vi "ROS_ParseMsg_r2.vi"(8 "Msg Package Path (blank)":path, 9 "Message Type":string, 11 "msg in":string) -> (1 "data":variant[](array[variant]), 3 "msg out":string)   [LabVIEW 2016]
doc: "Parses a ROS message based on the Message Type. Message Type must be a valid .txt file in the RosMessages directory."
uses:
  std_msgs/subs/parse_bool_scalar.vi
  std_msgs/subs/parse_i8_scalar.vi
  std_msgs/subs/parse_u8_scalar.vi
  std_msgs/subs/parse_i16_scalar.vi
  std_msgs/subs/parse_u16_scalar.vi
  std_msgs/subs/parse_i32_scalar.vi
  std_msgs/subs/parse_u32_scalar.vi
  std_msgs/subs/parse_i64_scalar.vi
  std_msgs/subs/parse_u64_scalar.vi
  std_msgs/subs/parse_float32_scalar.vi
  std_msgs/subs/parse_float64_scalar.vi
  std_msgs/subs/parse_string_scalar.vi
  std_msgs/subs/parse_time_scalar.vi
  std_msgs/subs/parse_duration_scalar.vi
panel:
  out "Data Types":string[](array[string])
  out "Data Names":string[](array[string])
  out "msg def":string
  out "Comments":string[](array[string])
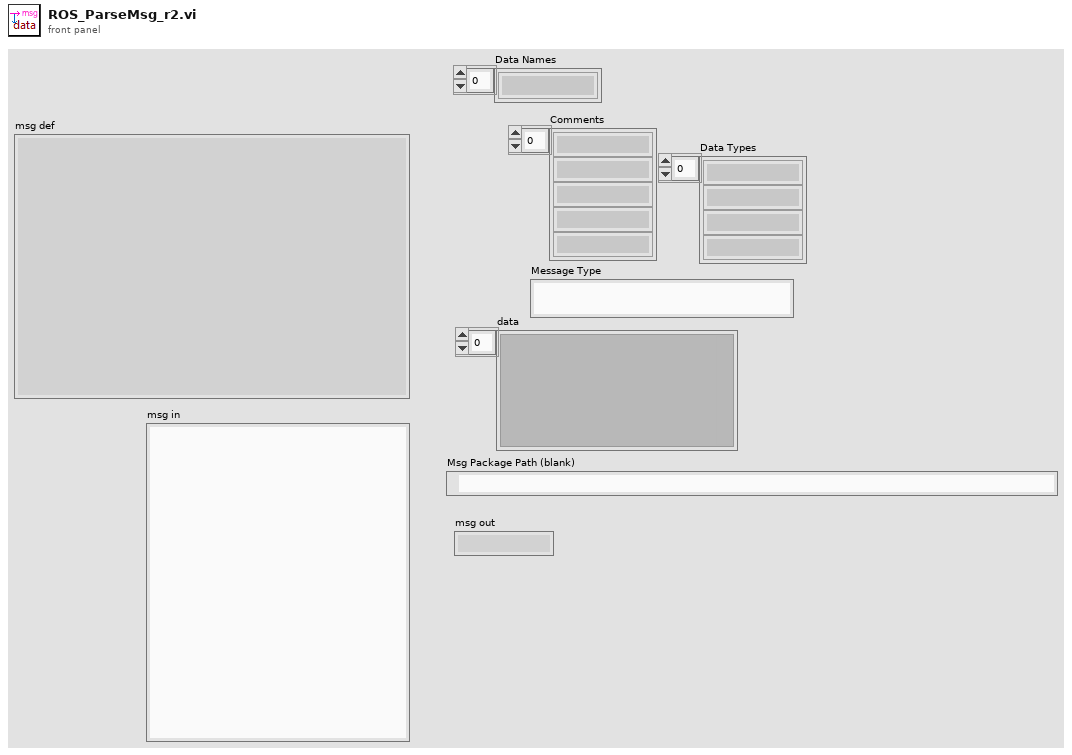
[diagram p1: front panel]
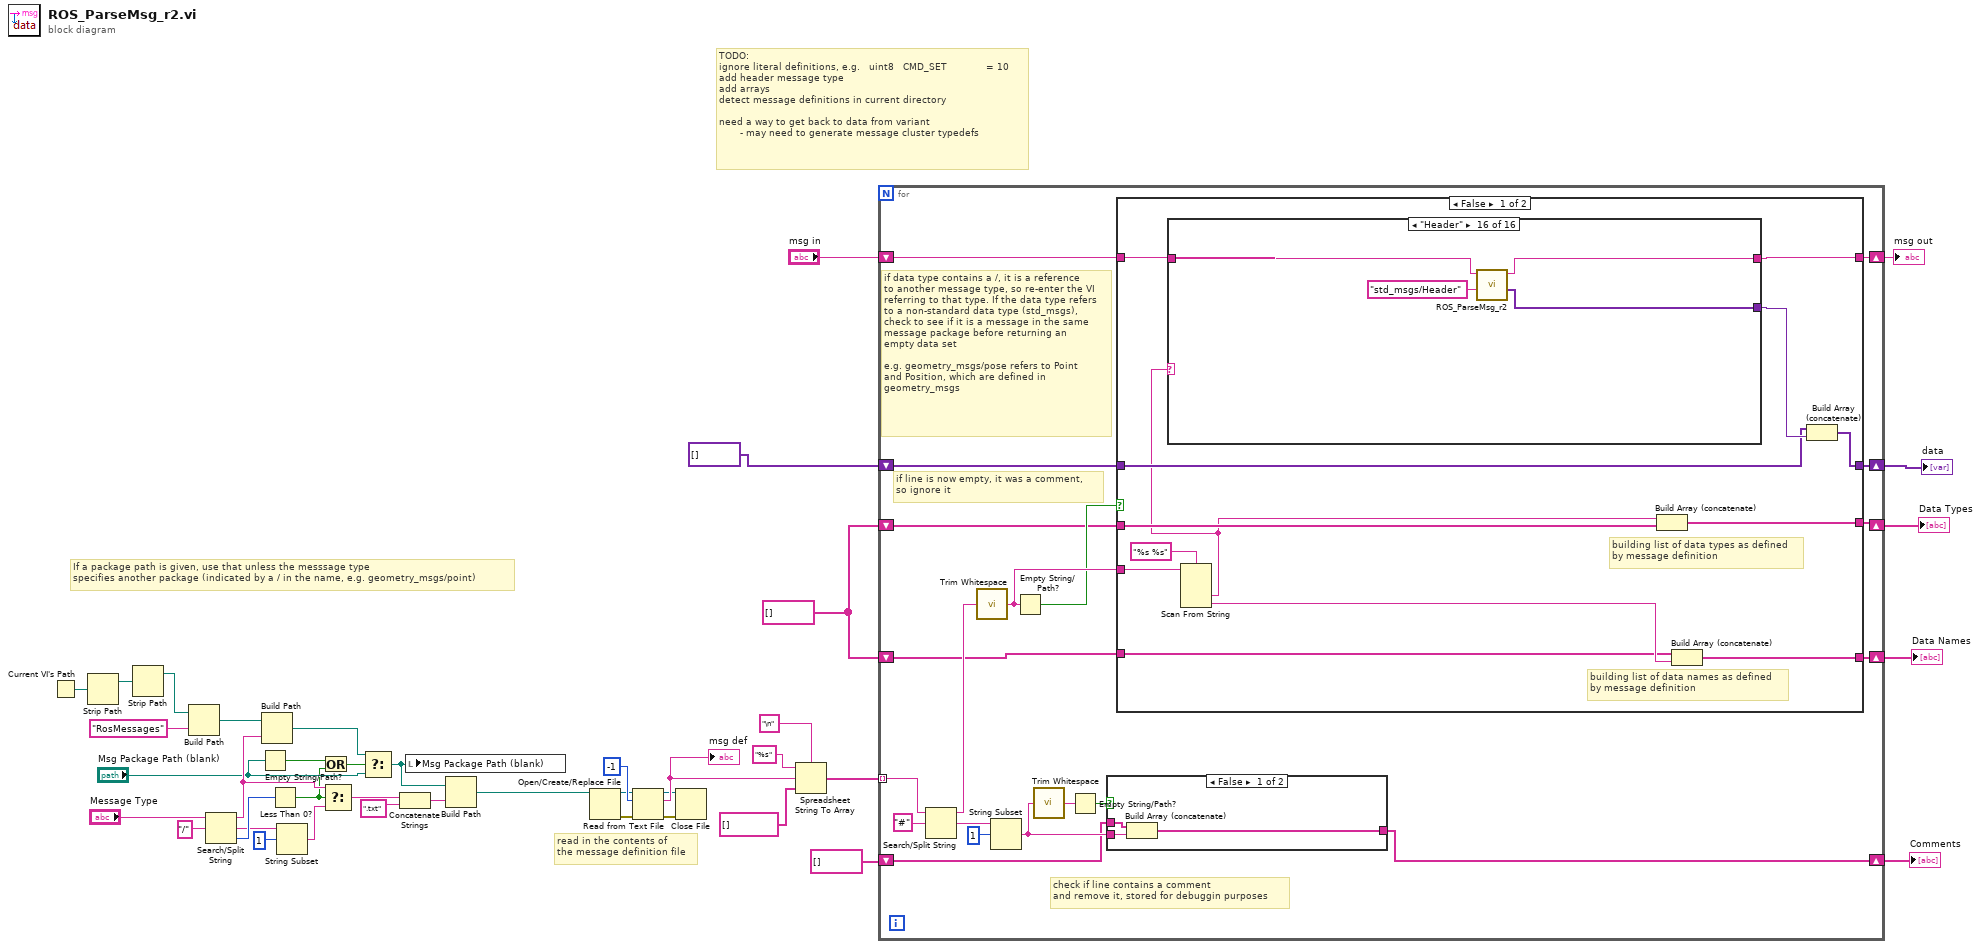
[diagram p0: block diagram]
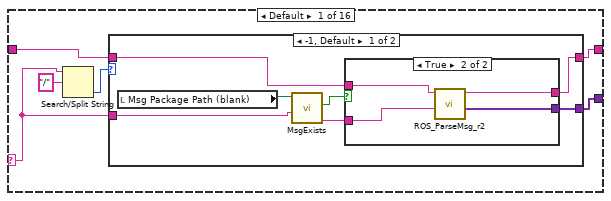
[diagram p2: hidden frame]
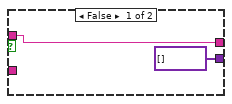
[diagram p3: hidden frame]
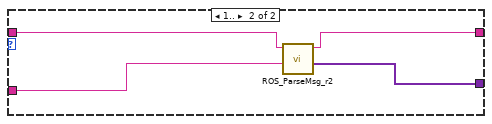
[diagram p4: hidden frame]
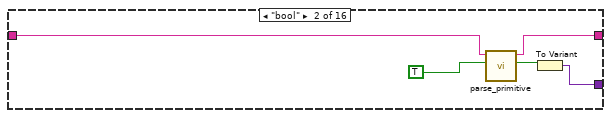
[diagram p5: hidden frame]
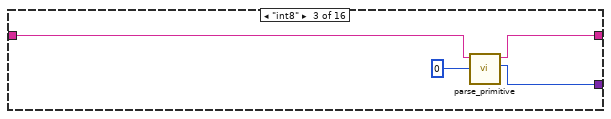
[diagram p6: hidden frame]
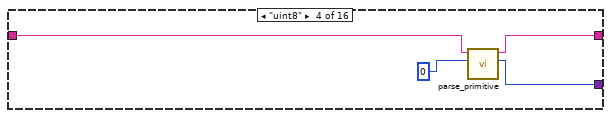
[diagram p7: hidden frame]
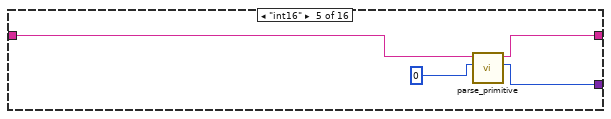
[diagram p8: hidden frame]
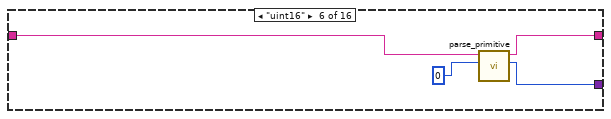
[diagram p9: hidden frame]
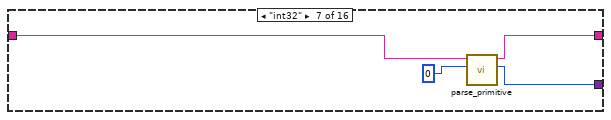
[diagram p10: hidden frame]
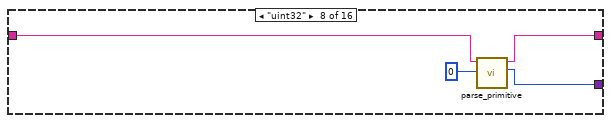
[diagram p11: hidden frame]
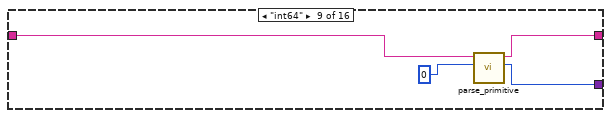
[diagram p12: hidden frame]
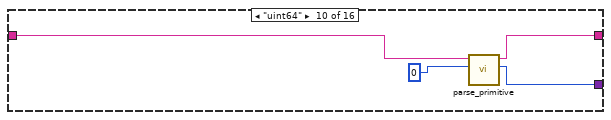
[diagram p13: hidden frame]
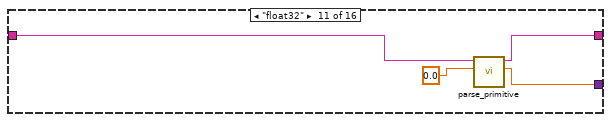
[diagram p14: hidden frame]
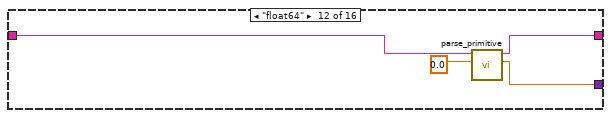
[diagram p15: hidden frame]
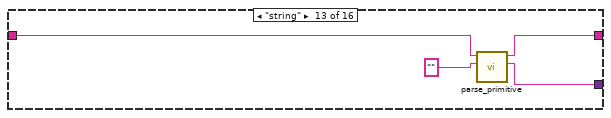
[diagram p16: hidden frame]
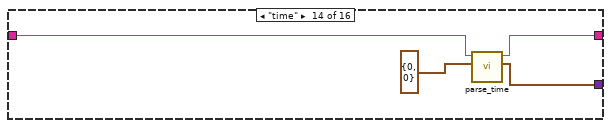
[diagram p17: hidden frame]
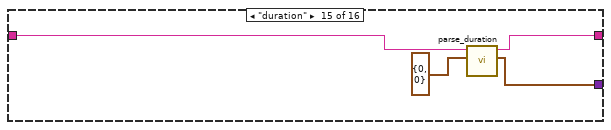
[diagram p18: hidden frame]
diagram:
  w25 = string[] []
  # "read in the contents of\nthe message definition file"
  # "If a package path is given, use that unless the messsage type\nspecifies another package (indicated by a / in the name, e.g. geometry_msgs/point)"
  # "TODO:\nignore literal definitions, e.g.   uint8   CMD_SET             = 10\nadd header message type\nadd arrays\ndetect message definitions in current directory\n\nneed a way to get back to data from variant\n       - may need to generate message cluster typedefs"
  n1 = Current VI's Path() -> (path=w24:path)
  n2 = Strip Path(path=w24) -> (stripped path=w23:path)  [unwired: 1 out]
  n3 = Strip Path(path=w23) -> (stripped path=w22:path)  [unwired: 1 out]
  n4 = Build Path(base path=w22, name or relative path="RosMessages") -> (appended path=w18:path)
  n5 = Search/Split String(string="Message Type", search string/char (-)="/") -> (substring before match=w13:string, match + rest of string=w11:string, offset of match=w14:i32)  [unwired: 1 in]
  n6 = Empty String/Path?(string/path="Msg Package Path (blank)") -> (empty?=w8:bool)
  n7 = Build Path(base path=w18, name or relative path=w13) -> (appended path=w6:path)
  n8 = Less Than 0?(x=w14) -> (x < 0?=w4:bool)
  n9 = String Subset(string=w11, offset (0)=1) -> (substring=w9:string)  [unwired: 1 in]
  n10 = Or(x=w8, y=w4) -> (x .or. y?=w5:bool)
  n11 = Select(t=w13, s=w4, f=w9) -> (s? t:f=w12:string)
  n12 = Select(t=w6, s=w5, f="Msg Package Path (blank)") -> (s? t:f=w15:path)
  n13 = Concatenate Strings(w12, ".txt" ("string")) -> (w17:string)
  n14 = local write "Msg Package Path (blank)"(w15) -> ()
  n15 = Build Path(base path=w15, name or relative path=w17) -> (appended path=w3:path)
  n16 = Open/Create/Replace File(file path (use dialog)=w3) -> (refnum out=w28:refnum<file>, error out=w29:errorcluster)  [unwired: 5 in, 1 out]
  n17 = Read from Text File(file (use dialog)=w28, count=-1, error in=w29) -> (refnum out=w31:refnum<file>, text=w32:string, error out=w30:errorcluster)  [unwired: 1 in, 1 out]
  "msg def" <- w32
  n18 = Close File(refnum=w31, error in=w30) -> ()  [unwired: 2 out]
  n19 = Spreadsheet String To Array(delimiter (Tab)="\n", format string="%s", spreadsheet string=w32, array type (2D Dbl)=string[] []) -> (array=w38:string[])
  n20 = for {
    tunnel: w38 -> [w60] mode=indexing
    shift-right: [w49] -> w2
    shift-left: variant[] [] -> [w50]
    shift-right: [w53] -> w37
    shift-left: string[] [] -> [w54]
    shift-right: [w51] -> w27
    shift-left: "msg in" -> [w52]
    shift-right: [w45] -> w1
    shift-left: w25 -> [w44]
    shift-right: [w43] -> w26
    shift-left: w25 -> [w42]
    # "if data type contains a /, it is a reference\nto another message type, so re-enter the VI\nreferring to that type. If the data type refers\nto a non-standard data type (std_msgs),\ncheck to see if it is a message in the same\nmessage package before returning an\nempty data set\n\ne.g. geometry_msgs/pose refers to Point\nand Position, which are defined in\ngeometry_msgs"
    # "if line is now empty, it was a comment,\nso ignore it"
    # "check if line contains a comment\nand remove it, stored for debuggin purposes"
    n21 = Search/Split String(string=w60, search string/char (-)="#") -> (substring before match=w48:string, match + rest of string=w59:string)  [unwired: 1 in, 1 out]
    n22 = call "Trim Whitespace.vi"("string"=w48) -> ("trimmed string"=w47:string)  [unwired: 1 in]
    n23 = String Subset(string=w59, offset (0)=1) -> (substring=w55:string)  [unwired: 1 in]
    n24 = Empty String/Path?(string/path=w47) -> (empty?=w46:bool)
    n25 = call "Trim Whitespace.vi"("string"=w55) -> ("trimmed string"=w57:string)  [unwired: 1 in]
    n26 = Empty String/Path?(string/path=w57) -> (empty?=w56:bool)
    n27 = case shown="False" w56 {
      tunnel: w55 -> [w165 _]
      tunnel: w54 -> [w164 w166]
      tunnel: [w163 w166] -> w53
      frame False {
        n28 = Build Array (concatenate)(w164, w165) -> (w163:string[])
      }
      frame True {
      }
    }
    n29 = case shown="False" w46 {
      tunnel: w52 -> [w74 w162]
      tunnel: [w73 w162] -> w51
      tunnel: w50 -> [w69 w161]
      tunnel: [w68 w161] -> w49
      tunnel: w47 -> [w71 _]
      tunnel: [w66 w160] -> w45
      tunnel: w44 -> [w65 w160]
      tunnel: [w64 w159] -> w43
      tunnel: w42 -> [w63 w159]
      frame False {
        # "building list of data names as defined\nby message definition"
        # "building list of data types as defined\nby message definition"
        n30 = Scan From String(format string="%s %s", input string=w71) -> (output 1=w62:string, output 2=w67:string)  [unwired: 4 in, 3 out]
        n31 = case shown="\"Header\"" w62 {
          selector: w62 -> [w75 _ _ _ _ _ _ _ _ _ _ _ _ _ _ _]
          tunnel: w74 -> [w80 w101 w106 w110 w114 w118 w122 w125 w130 w134 w138 w142 w145 w150 w154 w158]
          tunnel: [w77 w100 w105 w108 w113 w116 w120 w124 w129 w133 w136 w140 w144 w148 w153 w155] -> w73
          tunnel: [w78 w98 w103 w107 w111 w115 w119 w123 w127 w131 w135 w139 w143 w147 w152 w156] -> w70
          frame Default {
            n32 = Search/Split String(string=w75, search string/char (-)="/") -> (offset of match=w79:i32)  [unwired: 1 in, 2 out]
            n33 = case shown="-1, Default" w79 {
              tunnel: w80 -> [w85 w95]
              tunnel: [w83 w97] -> w78
              tunnel: [w84 w96] -> w77
              tunnel: w75 -> [w82 w94]
              frame -1, Default {
                n34 = local read "Msg Package Path (blank)"() -> (w81:path)
                n35 = call "MsgExists.vi"("Msg Type"=w82, "Msg Path"=w81) -> ("Package/Msg"=w86:string, "Msg Exists?"=w87:bool)  [unwired: 8 in]
                n36 = case shown="True" w87 {
                  tunnel: w86 -> [_ w93]
                  tunnel: w85 -> [w89 w92]
                  tunnel: [w89 w91] -> w84
                  tunnel: [variant[] [] ("data") w90] -> w83
                  frame False {
                  }
                  frame True {
                    n37 = call "ROS_ParseMsg_r2.vi"("Message Type"=w93, "msg in"=w92) -> ("data"=w90:variant[], "msg out"=w91:string)  [unwired: 8 in]
                  }
                }
              }
              frame 1.. {
                n38 = call "ROS_ParseMsg_r2.vi"("Message Type"=w94, "msg in"=w95) -> ("data"=w97:variant[], "msg out"=w96:string)  [unwired: 8 in]
              }
            }
          }
          frame "bool" {
            n39 = call-poly "parse_primitive.vi"("type"=TRUE, "msg in"=w101) -> ("bool"=w99:bool, "msg out"=w100:string)  [unwired: 3 in, 1 out]
            n40 = To Variant(anything=w99) -> (Variant=w98:variant)
          }
          frame "int8" {
            n41 = call-poly "parse_primitive.vi"("type"=i8 0, "msg in"=w106) -> ("number"=w103:i8, "msg out"=w105:string)  [unwired: 3 in, 1 out]
          }
          frame "uint8" {
            n42 = call-poly "parse_primitive.vi"("type"=u8 0, "msg in"=w110) -> ("number"=w107:u8, "msg out"=w108:string)  [unwired: 3 in, 1 out]
          }
          frame "int16" {
            n43 = call-poly "parse_primitive.vi"("type"=i16 0, "msg in"=w114) -> ("number"=w111:i16, "msg out"=w113:string)  [unwired: 3 in, 1 out]
          }
          frame "uint16" {
            n44 = call-poly "parse_primitive.vi"("type"=u16 0, "msg in"=w118) -> ("number"=w115:u16, "msg out"=w116:string)  [unwired: 3 in, 1 out]
          }
          frame "int32" {
            n45 = call-poly "parse_primitive.vi"("type"=0, "msg in"=w122) -> ("number"=w119:i32, "msg out"=w120:string)  [unwired: 3 in, 1 out]
          }
          frame "uint32" {
            n46 = call-poly "parse_primitive.vi"("type"=u32 0, "msg in"=w125) -> ("number"=w123:u32, "msg out"=w124:string)  [unwired: 3 in, 1 out]
          }
          frame "int64" {
            n47 = call-poly "parse_primitive.vi"("type"=i64 0, "msg in"=w130) -> ("number"=w127:i64, "msg out"=w129:string)  [unwired: 3 in, 1 out]
          }
          frame "uint64" {
            n48 = call-poly "parse_primitive.vi"("type"=u64 0, "msg in"=w134) -> ("number"=w131:u64, "msg out"=w133:string)  [unwired: 3 in, 1 out]
          }
          frame "float32" {
            n49 = call-poly "parse_primitive.vi"("type"=sgl 0.0, "msg in"=w138) -> ("number"=w135:sgl, "msg out"=w136:string)  [unwired: 3 in, 1 out]
          }
          frame "float64" {
            n50 = call-poly "parse_primitive.vi"("type"=0.0, "msg in"=w142) -> ("number"=w139:dbl, "msg out"=w140:string)  [unwired: 3 in, 1 out]
          }
          frame "string" {
            n51 = call-poly "parse_primitive.vi"("type"="" ("delimiter (Tab)"), "msg in"=w145) -> ("string"=w143:string, "msg out"=w144:string)  [unwired: 3 in, 1 out]
          }
          frame "time" {
            n52 = call-poly "parse_time.vi"("type"=cluster{"secs":i32, "nsecs":i32} {"secs"=0, "nsecs"=0}, "msg in"=w150) -> ("Time"=w147:cluster{"secs":i32, "nsecs":i32}, "msg out"=w148:string)  [unwired: 3 in, 1 out]
          }
          frame "duration" {
            n53 = call-poly "parse_duration.vi"("type"=cluster{"secs":i32, "nsecs":i32} {"secs"=0, "nsecs"=0}, "msg in"=w154) -> ("Duration"=w152:cluster{"secs":i32, "nsecs":i32}, "msg out"=w153:string)  [unwired: 3 in, 1 out]
          }
          frame "Header" {
            n54 = call "ROS_ParseMsg_r2.vi"("Message Type"="std_msgs/Header", "msg in"=w158) -> ("data"=w156:variant[], "msg out"=w155:string)  [unwired: 8 in]
          }
        }
        n55 = Build Array (concatenate)(w62, w63) -> (w64:string[])
        n56 = Build Array (concatenate)(w65, w67) -> (w66:string[])
        n57 = Build Array (concatenate)(w69, w70) -> (w68:variant[])
      }
      frame True {
      }
    }
  }
  "Comments" <- w37
  "msg out" <- w27
  "data" <- w2
  "Data Names" <- w1
  "Data Types" <- w26
